vi "NewDataAdded Event Callback.vi"(4 "User Parameter":T1, 5 "Event Data":cluster{"sender":refnum<k24>, "e":refnum<k24>}, 6 "Control Ref":refnum<k24>, 7 "Event Common Data":T2) -> ()   [LabVIEW 2020]
uses:
  C:/Utils/LabVIEWNETSDK - Class/PalmSens/Libraries/PalmSens.Core.Simplified.dll
  Libraries/PalmSens.Core.Simplified.dll
  C:/Utils/LabVIEWNETSDK - Class/PalmSens/Libraries/PalmSens.Core.dll
  Libraries/PalmSens.Core.dll
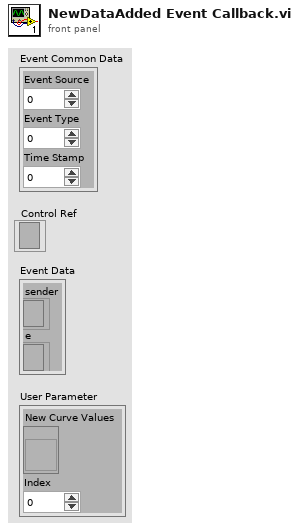
[diagram p1: front panel]
types:
  T1 = cluster{"New Curve Values":refnum<vi>, "Index":i16}
  T2 = cluster{"Event Source":i32, "Event Type":u32, "Time Stamp":u32}
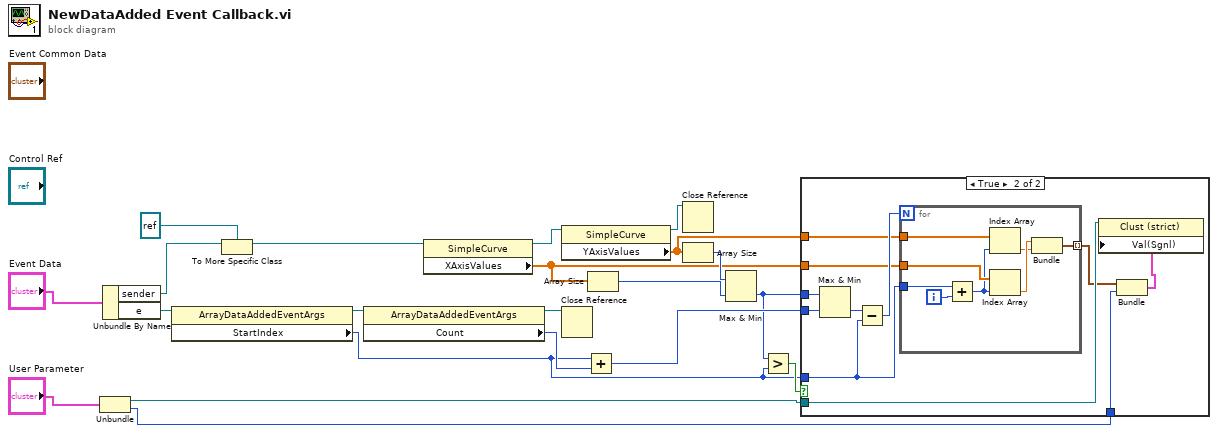
[diagram p0: block diagram]
diagram:
  n1 = Unbundle("User Parameter") -> ("New Curve Values"=w4:refnum<vi>, "Index"=w3:i16)
  n2 = Unbundle By Name("Event Data") -> ("sender"=w19:refnum<k24>, "e"=w21:refnum<k24>)
  n3 = property class="ArrayDataAddedEventArgs"(reference=w21) -> (reference out=w20:refnum<k24>, "StartIndex"=w7:i32)  [unwired: 1 in, 1 out]
  n4 = To More Specific Class(target class=refnum<k24> refnum, reference=w19) -> (specific class reference=w17:refnum<k24>)  [unwired: 1 in, 1 out]
  n5 = property class="ArrayDataAddedEventArgs"(reference=w20) -> (reference out=w5:refnum<k24>, "Count"=w15:i32)  [unwired: 1 in, 1 out]
  n6 = property class="SimpleCurve"(reference=w17) -> (reference out=w16:refnum<k24>, "XAxisValues"=w9:dbl[])  [unwired: 1 in, 1 out]
  n7 = property class="SimpleCurve"(reference=w16) -> (reference out=w6:refnum<k24>, "YAxisValues"=w8:dbl[])  [unwired: 1 in, 1 out]
  n8 = Close Reference(reference=w5) -> ()  [unwired: 1 in, 1 out]
  n9 = Add(x=w7, y=w15) -> (x+y=w12:i32)
  n10 = Array Size(array=w9) -> (size(s)=w13:i32)
  n11 = Close Reference(reference=w6) -> ()  [unwired: 1 in, 1 out]
  n12 = Array Size(array=w8) -> (size(s)=w14:i32)
  n13 = Max & Min(x=w14, y=w13) -> (min(x,y)=w10:i32)  [unwired: 1 out]
  n14 = Greater?(x=w10, y=w7) -> (0:w11:bool)
  n15 = case shown="True" w11 {
    tunnel: w12 -> [_ w32]
    tunnel: w10 -> [_ w31]
    tunnel: w7 -> [_ w27]
    tunnel: w9 -> [_ w28]
    tunnel: w8 -> [_ w26]
    tunnel: w4 -> [_ w25]
    tunnel: w3 -> [_ w23]
    frame False {
    }
    frame True {
      n16 = Max & Min(x=w31, y=w32) -> (min(x,y)=w30:i32)  [unwired: 1 out]
      n17 = Subtract(x=w30, y=w27) -> (x-y=w29:i32)
      n18 = for {
        N: w29 -> [_]
        tunnel: w28 -> [w40]
        tunnel: w27 -> [w38]
        tunnel: w26 -> [w36]
        tunnel: [w33] -> w24 mode=indexing
        i -> [w39]
        n19 = Add(x=w38, y=w39) -> (x+y=w35:i32)
        n20 = Index Array(array=w36, index=w35) -> (element=w34:dbl)
        n21 = Index Array(array=w40, index=w35) -> (element=w37:dbl)
        n22 = Bundle(w37, w34) -> (w33:cluster{dbl, dbl})  [unwired: 1 in]
      }
      n23 = Bundle(w24, "Index"=w23) -> (w22:cluster{cluster{dbl, dbl}[], "Index":i16})  [unwired: 1 in]
      n24 = property class="Clust (strict)"(reference=w25, "Val(Sgnl)"=w22) -> ()  [unwired: 1 in, 2 out]
    }
  }
